vi "GenNet Receive UDP Message.vi"(6 "timeout [ms]":i32=1000, 8 "error in (no error)":errorcluster, 10 "Max Byte Size":i32, 11 "UDP Network Connection in":refnum<k16>) -> (0 "error out":errorcluster, 2 "Message Data":variant, 3 "UDP Network Connection out":refnum<k16>)   [LabVIEW 2022 SP3, in "hse-gennet.lvlib"]
doc: "Receives a message sent by a GenNet-Client module. The first 4 bytes of the message contain the lenght of the actual data sent. The received message is converted to a variant.\n\n____\nHAMPEL SOFTWARE ENGINEERING v3.8.0 (2023-12-18 14:41)"
uses:
  hse-gennet.lvlib
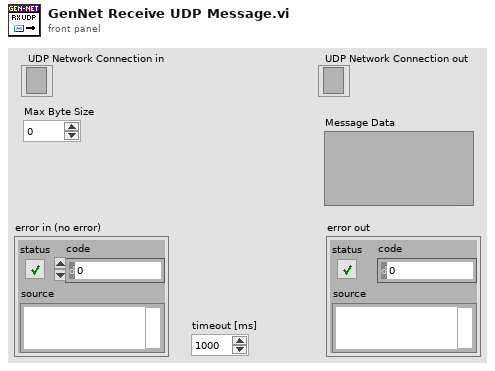
[diagram p1: front panel]
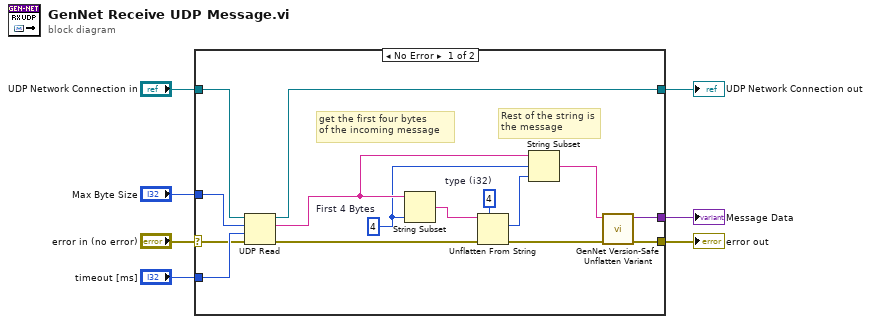
[diagram p0: block diagram]
diagram:
  n1 = case shown="No Error" "error in (no error)" {
    selector: "error in (no error)" -> [w17 w23]
    tunnel: "UDP Network Connection in" -> [w19 w24]
    tunnel: [w9 w24] -> w3
    tunnel: "timeout [ms]" -> [w18 _]
    tunnel: [w22 w23] -> w6
    tunnel: [w21 _] -> w5
    tunnel: "Max Byte Size" -> [w8 _]
    frame No Error {
      w20 = 4  # type (i32)
      w10 = 4  # First 4 Bytes
      # "Rest of the string is the message"
      # "get the first four bytes\nof the incoming message"
      n2 = UDP Read(connection ID=w19, max size (548)=w8, timeout ms (25000)=w18, 8:w17) -> (data out=w13:string, error out=w16:errorcluster, 3:w9:refnum<k16>)  [unwired: 2 out]
      n3 = String Subset(string=w13, length (rest)=w10) -> (substring=w15:string)  [unwired: 1 in]
      n4 = Unflatten From String(type=w20, binary string=w15, error in (no error)=w16) -> (value=w14:i32, error out=w11:errorcluster)  [unwired: 2 in, 1 out]
      n5 = String Subset(string=w13, offset (0)=w10, length (rest)=w14) -> (substring=w12:string)
      n6 = call "GenNet Version-Safe Unflatten Variant.vi"("error in"=w11, "Flattened Data"=w12) -> ("error out"=w22:errorcluster, "Message Data"=w21:variant)  [unwired: 8 in]
    }
    frame Error {
    }
  }
  "error out" <- w6
  "Message Data" <- w5
  "UDP Network Connection out" <- w3
